vi "Lego1.vi"() -> ()   [LabVIEW 2022 SP3]
panel:
  in  "stop":bool
  out "Frequency offset":dbl
  out "Modulation parameter":T1
  out "XY Graph":cdb[](graph)
  out "string 2":string
  out "Led1":bool
  out "element":u8
  out "output byte stream":u8[](array[numeric])
  out "size(s)":i32
  out "SIG valid?":bool
  out "error out":errorcluster
  out "created new?":bool
  out "Numeric 2":i32
  out "x .or. y?":bool
  out "USRP CoercedParamters":T2={"coerced IQ rate"=100000.0, "coerced carrier frequency"=100000.0, "coerced gain"=0.0} {"coerced gain" format="%#_6f"; "coerced carrier frequency" format="%#_6p"; "coerced IQ rate" format="%#_6p"}
  in  "Trigger level":dbl=0.005 format="%f"
  in  "error in (no error)":errorcluster
  in  "USRP ControledParameters":T3={"active antenna"="RX1", "gain"=10.0, "carrier frequency"=2400000000.0, "IQ rate"=2000000.0} {"IQ rate" format="%#_6p"; "carrier frequency" format="%#_6p"; "gain" format="%#_6f"}
  in  "device names":refnum<k15>="RIO0"
  out "Boolean 2":bool
  out "Boolean":bool
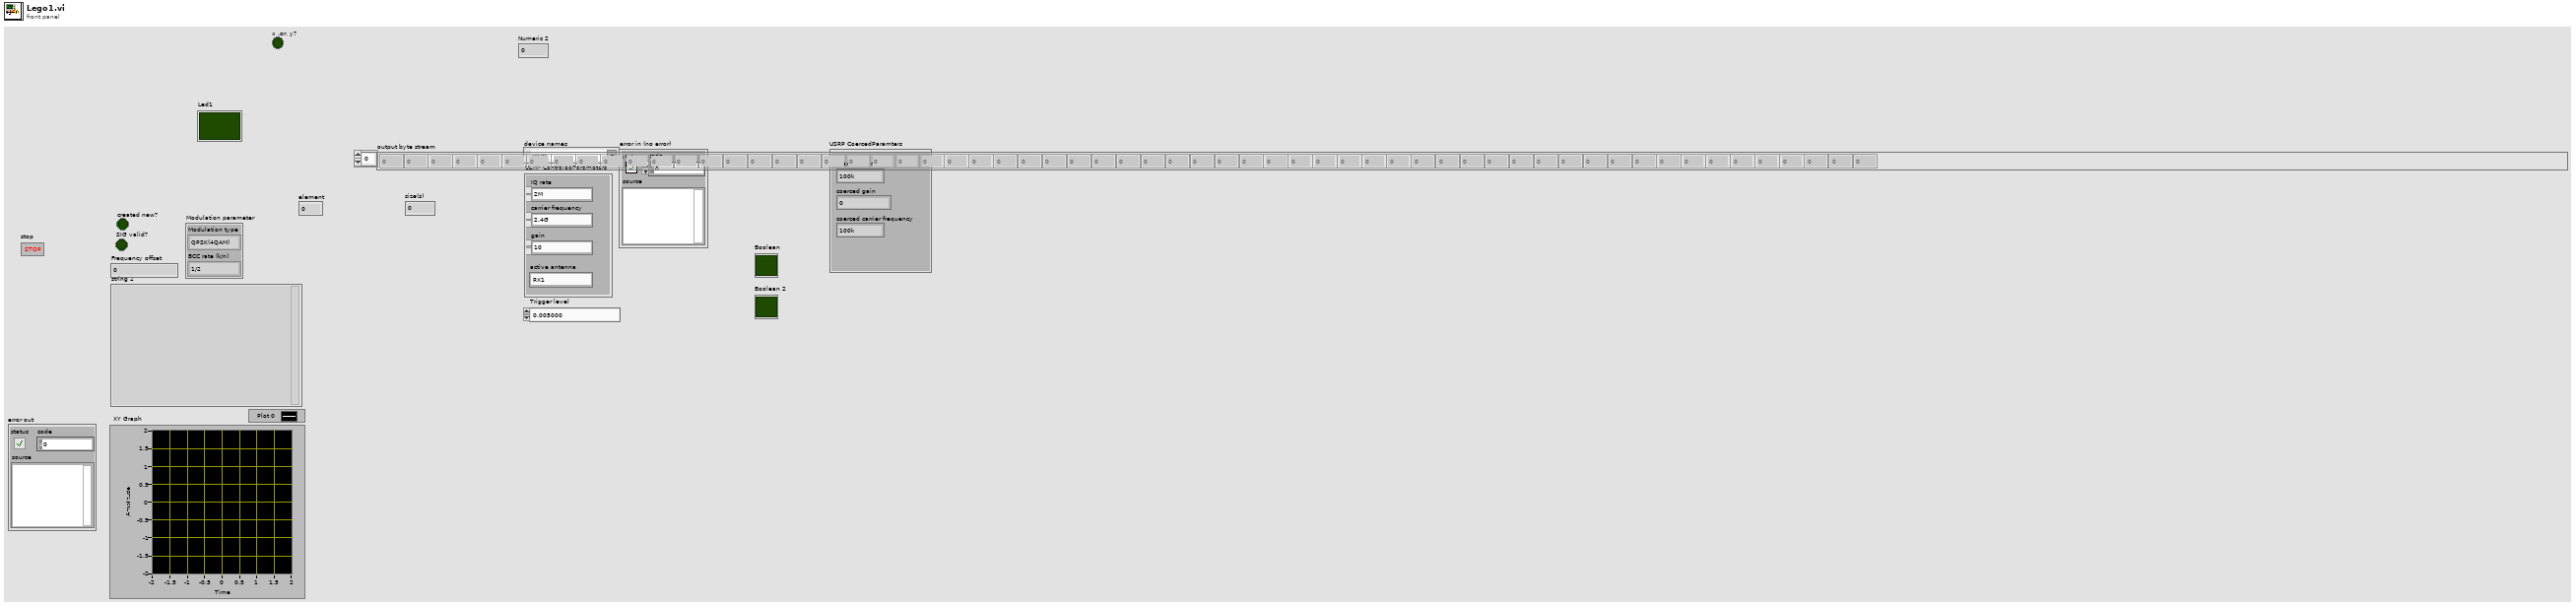
[diagram p1: front panel]
types:
  T1 = cluster{"Modulation type":enum16{"QPSK(4QAM)", "64QAM", "16QAM", "BPSK"}, "BCC rate (k/n)":enum16{"1/2", "2/3", "3/4"}}
  T2 = cluster{"coerced IQ rate":dbl, "coerced carrier frequency":dbl, "coerced gain":dbl}
  T3 = cluster{"active antenna":string, "gain":dbl, "carrier frequency":dbl, "IQ rate":dbl}
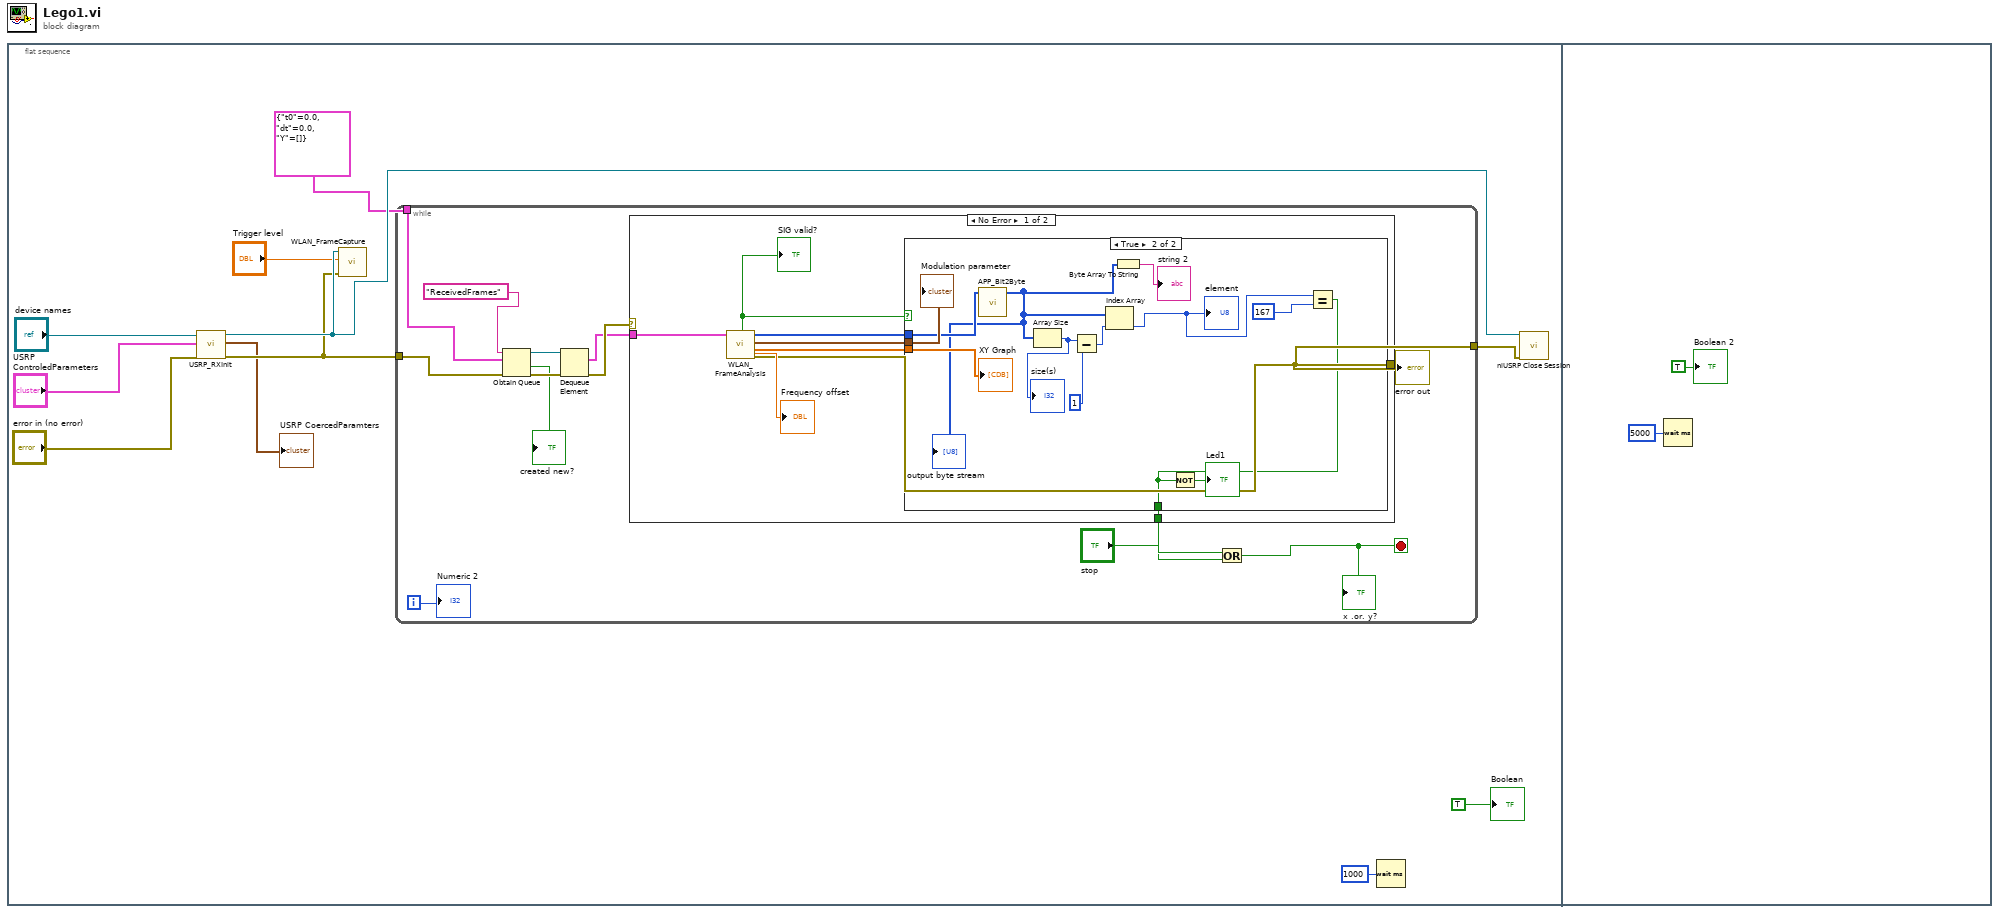
[diagram p0: block diagram]
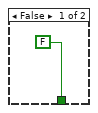
[diagram p2: hidden frame]
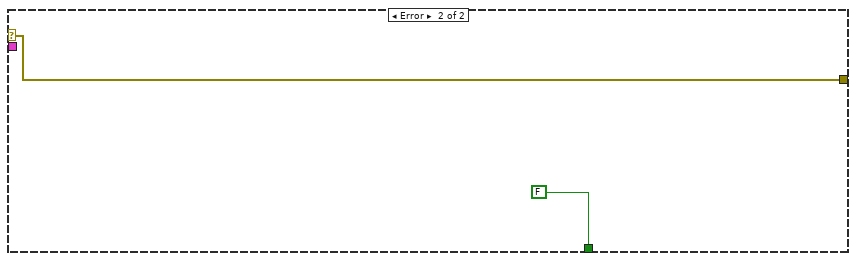
[diagram p3: hidden frame]
diagram:
  n1 = flat-sequence {
    frame #0 {
      n2 = call "USRP_RXInit.vi"("device names"="device names", "USRP ControledParameters"="USRP ControledParameters", "error in (no error)"="error in (no error)") -> ("session handle out"=w9:refnum<k15>, "USRP CoercedParamters"=→"USRP CoercedParamters":T2, "error out"=w6:errorcluster)  [unwired: 5 in]
      n3 = call "WLAN_FrameCapture.vi"("error in (no error)"=w6, "Trigger level"="Trigger level", "session handle"=w9) -> ()  [unwired: 8 in]
      n4 = while {
        tunnel: w6 -> [w23]
        tunnel: cluster{"t0":dbl, "dt":dbl, "Y":cdb[]} {"t0"=0.0, "dt"=0.0, "Y"=[]} ("data") -> [w24]
        tunnel: [w16] -> w8
        i -> [w12]
        stop <- w14 stop-if-true
        n5 = Obtain Queue(name (unnamed)="ReceivedFrames", element data type=w24, error in (no error)=w23) -> (queue out=w22:refnum<queue>, created new?=→"created new?":bool, error out=w19:errorcluster)  [unwired: 2 in]
        n6 = Dequeue Element(queue=w22, error in (no error)=w19) -> (element=w20:cluster{"t0":dbl, "dt":dbl, "Y":cdb[]}, error out=w21:errorcluster)  [unwired: 1 in, 2 out]
        n7 = case shown="No Error" w21 {
          selector: w21 -> [_ w47]
          tunnel: w20 -> [w26 _]
          tunnel: [w27 w47] -> w16
          tunnel: [w25 FALSE] -> w13
          frame No Error {
            n8 = call "WLAN_FrameAnalysis.vi"("input cluster"=w26) -> ("error out"=w27:errorcluster, "Constellation"=w29:cdb[], "Modulation parameter"=w28:T1, "output bits"=w30:i8[], "Frequency offset"=→"Frequency offset":dbl, "SIG valid?"=w31:bool)  [unwired: 5 in]
            "SIG valid?" <- w31
            n9 = case shown="True" w31 {
              tunnel: w30 -> [_ w42]
              tunnel: w29 -> [_ w44]
              tunnel: w28 -> [_ w45]
              tunnel: [FALSE w34] -> w25
              frame False {
              }
              frame True {
                n10 = call "APP_Bit2Byte.vi"("input bit stream"=w42) -> ("output byte stream"=w41:u8[])  [unwired: 10 in]
                "output byte stream" <- w41
                n11 = Array Size(array=w41) -> (size(s)=w39:i32)
                "size(s)" <- w39
                n12 = Subtract(x=w39, y=1) -> (x-y=w38:i32)
                n13 = Index Array(array=w41, index=w38) -> (element=w36:u8)
                "element" <- w36
                n14 = Byte Array To String(unsigned byte array=w41) -> (string=→"string 2":string)
                n15 = Equal?(x=w36, y=u8 167) -> (x = y?=w34:bool)
                n16 = Not(x=w34) -> (.not. x?=→"Led1":bool)
                "Modulation parameter" <- w45
                "XY Graph" <- w44
              }
            }
          }
          frame Error {
          }
        }
        "error out" <- w16
        n17 = Or(x="stop", y=w13) -> (x .or. y?=w14:bool)
        "x .or. y?" <- w14
        "Numeric 2" <- w12
      }
      n18 = Wait (ms)(milliseconds to wait=u32 1000) -> ()  [unwired: 1 out]
      n19 = call <instrlib>:"niUSRP Close Session.vi"("session handle"=w9, "error in (no error)"=w8) -> ()  [unwired: 13 in, 1 out]
      "Boolean" <- TRUE ("Boolean")
    }
    frame #1 {
      n20 = Wait (ms)(milliseconds to wait=u32 5000) -> ()  [unwired: 1 out]
      "Boolean 2" <- TRUE ("Boolean 2")
    }
  }
